vi "Create_Trajectory_Field_Crop_and_Scale.vi"(4 "Field Y Ft":dbl=27.0 format="%#_13g", 5 "Disp Y Size Pixel":i32=580, 6 "Field X Ft":dbl=54.0 format="%#_13g", 7 "Disp X Size Pixel":i32=1160, 9 "Field Image":T1, 10 "field Info":T2, 11 "Display Image":T1) -> (2 "FIeld Image Out":T1, 3 "Disp Image Out":T1)   [LabVIEW 2019]
uses:
  TrajectoryUtils_Field_Info.ctl
  <vilib>/vision/Image Controls.llb/IMAQ Image.ctl
  <vilib>/vision/NI_Vision_Development_Module.lvlib
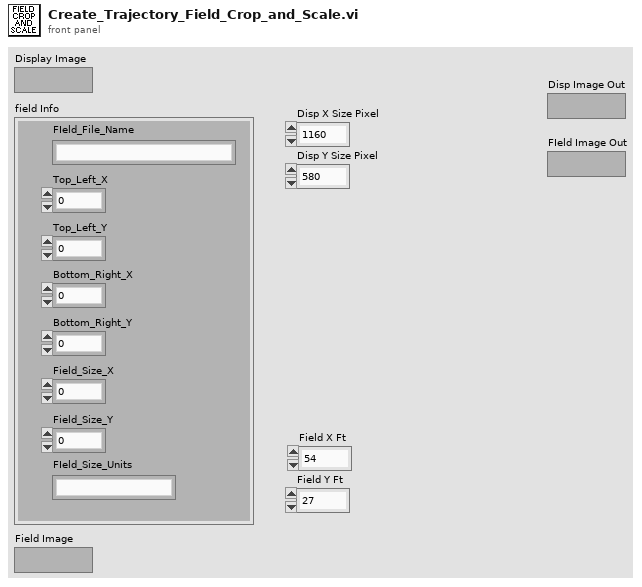
[diagram p1: front panel]
types:
  T1 = typedef "IMAQ Image.ctl" = refnum<image>
  T2 = typedef "TrajectoryUtils_Field_Info.ctl" = cluster{"FIeld_File_Name":string, "Top_Left_X":i32, "Top_Left_Y":i32, "Bottom_Right_X":i32, "Bottom_Right_Y":i32, "Field_Size_X":dbl, "Field_Size_Y":dbl, "FIeld_Size_Units":string}
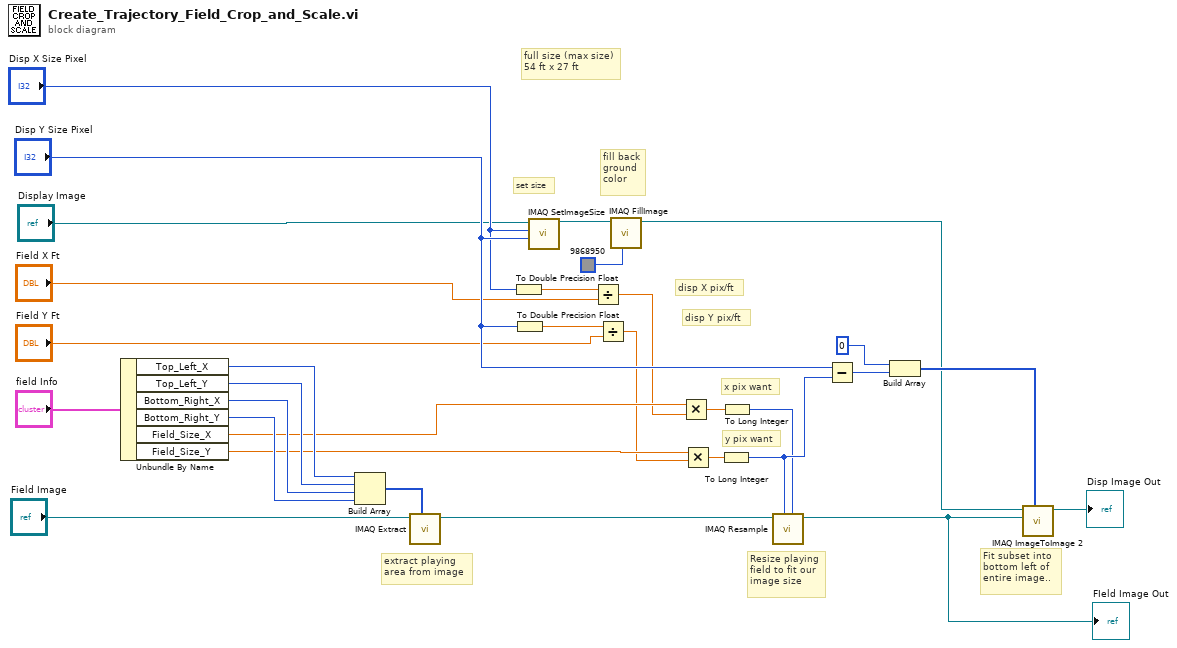
[diagram p0: block diagram]
diagram:
  # "Resize playing\nfield to fit our\nimage size"
  # "disp Y pix/ft"
  # "extract playing \narea from image"
  # "y pix want"
  # "x pix want"
  # "disp X pix/ft"
  # "fill back\nground\ncolor"
  # "set size"
  # "Fit subset into\nbottom left of \nentire image.."
  # "full size (max size)\n54 ft x 27 ft"
  n1 = Unbundle By Name("field Info") -> ("Top_Left_X"=w28:i32, "Top_Left_Y"=w29:i32, "Bottom_Right_X"=w30:i32, "Bottom_Right_Y"=w31:i32, "Field_Size_X"=w24:dbl, "Field_Size_Y"=w25:dbl)
  n2 = Build Array(w28, w29, w30, w31) -> (w2:i32[])
  n3 = call "IMAQ Extract"("Optional Rectangle"=w2, "Image Src"="Field Image") -> ("Image Dst Out"=w13:T1)  [unwired: 8 in, 1 out]
  n4 = To Double Precision Float(number="Disp X Size Pixel") -> (double precision float=w7:dbl)
  n5 = To Double Precision Float(number="Disp Y Size Pixel") -> (double precision float=w8:dbl)
  n6 = call "IMAQ SetImageSize"("Y Resolution"="Disp Y Size Pixel", "X Resolution"="Disp X Size Pixel", "Image"="Display Image") -> ("Image Out"=w4:T1)  [unwired: 2 in, 1 out]
  n7 = Divide(x=w7, y="Field X Ft") -> (x/y=w11:dbl)
  n8 = Divide(x=w8, y="Field Y Ft") -> (x/y=w12:dbl)
  n9 = call "IMAQ FillImage"("Color Pixel Value"=u32 9868950, "Image"=w4) -> ("Image Out"=w17:T1)  [unwired: 8 in, 1 out]
  n10 = Multiply(x=w24, y=w11) -> (x*y=w15:dbl)
  n11 = Multiply(x=w25, y=w12) -> (x*y=w16:dbl)
  n12 = To Long Integer(number=w16) -> (32bit integer=w20:i32)
  n13 = To Long Integer(number=w15) -> (32bit integer=w14:i32)
  n14 = call "IMAQ Resample"("X Resolution"=w14, "Y Resolution"=w20, "Image Src"=w13) -> ("Image Dst Out"=w21:T1)  [unwired: 7 in, 1 out]
  "FIeld Image Out" <- w21
  n15 = Subtract(x="Disp Y Size Pixel", y=w20) -> (x-y=w26:i32)
  n16 = Build Array(0, w26) -> (w22:i32[])
  n17 = call "IMAQ ImageToImage 2"("Offset Left/Top"=w22, "Image Src (Small)"=w21, "Image Src (Large)"=w17) -> ("Image Dst Out"=→"Disp Image Out":T1)  [unwired: 7 in, 1 out]
